vi "getScriptInfo.vi"(8 "error in (no error)":errorcluster, 11 "DataPointScript.lvclass in":refnum<class "DataPointScript.lvclass">) -> (0 "error out":errorcluster, 2 "Script info":string, 3 "DataPointScript.lvclass out":refnum<class "DataPointScript.lvclass">)   [LabVIEW 2009, in "Tools.lvlib" / "Scripting.lvlib" / "DataPointScript.lvclass"]
uses:
  DataPointScript.lvclass
  DataPointScript.lvclass/DataPointScript.ctl
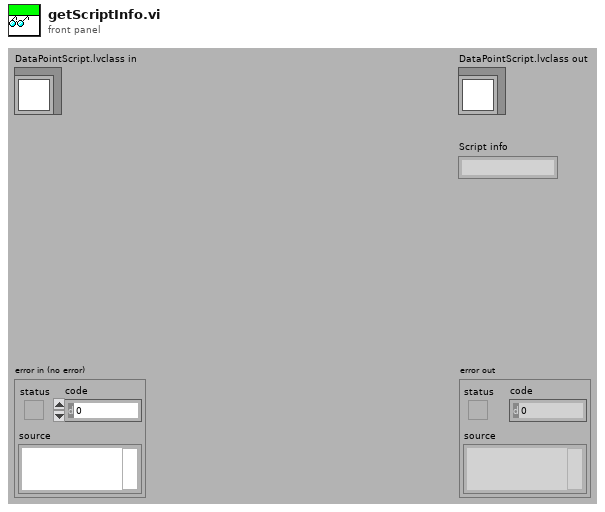
[diagram p1: front panel]
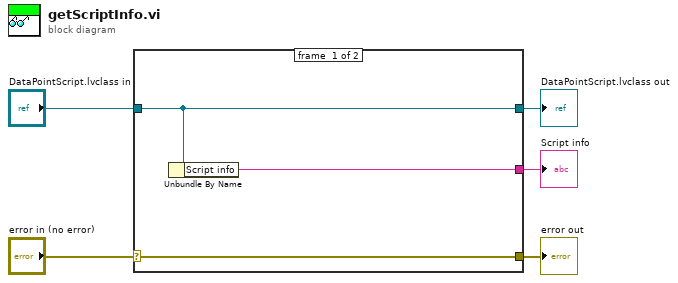
[diagram p0: block diagram]
diagram:
  n1 = case shown="No Error" "error in (no error)" {
    selector: "error in (no error)" -> [w8 w9]
    tunnel: [w8 w9] -> w4
    tunnel: [w7 w10] -> w2
    tunnel: "DataPointScript.lvclass in" -> [w7 w10]
    tunnel: [w6 _] -> w1
    frame #0 {
      n2 = Unbundle By Name(w7) -> ("Script info"=w6:string)
    }
    frame #1 {
    }
  }
  "error out" <- w4
  "DataPointScript.lvclass out" <- w2
  "Script info" <- w1
